vi "testing_cw_sweep.vi"() -> ()   [LabVIEW 2015, in "Tausand AB1000.lvlib"]
uses:
  <instrlib>/Tausand AB1000/Tausand AB1000.lvlib
  <instrlib>/Tausand AB1000/Public/Controls/deviceTypeRing.ctl
  <instrlib>/Tausand AB1000/Public/Controls/counters4ch.ctl
  <instrlib>/Tausand AB1000/Public/Controls/channelRing.ctl
panel:
  in  "device type (any)":T1 items=["any"=0, "AB1002"=1002, "AB1004"=1004, "AB1502"=1502, "AB1504"=1504, "AB1902"=1902, "AB1904"=1904, "AB2002"=2002, "AB2004"=2004, "AB2502"=2502, "AB2504"=2504, "AB2902"=2902, "AB2904"=2904]
  out "tausand values":u32[][](array[numeric])
  in  "delay D (ns)":u32
  in  "delay C (ns)":u32
  in  "delay B (ns)":u32
  in  "delay A (ns)":u32
  out "i case":i32
  out "total cases":i32
  in  "Stop Button":bool
  out "coinc Chart":T2(graph)
  out "current values":T3
  in  "sampling (ms)":u32=1000
  out "i cw":i32
  out "device type":T1 items=["any"=0, "AB1002"=1002, "AB1004"=1004, "AB1502"=1502, "AB1504"=1504, "AB1902"=1902, "AB1904"=1904]
  out "cw array":u32[](array[numeric])
  in  "step cw":u32=1
  in  "max cw":u32=10
  in  "min cw":u32=1
  out "current cw (ns)":u32
  in  "VISA resource name":refnum<visa-resource-name>
  # "case"
  # "out of"
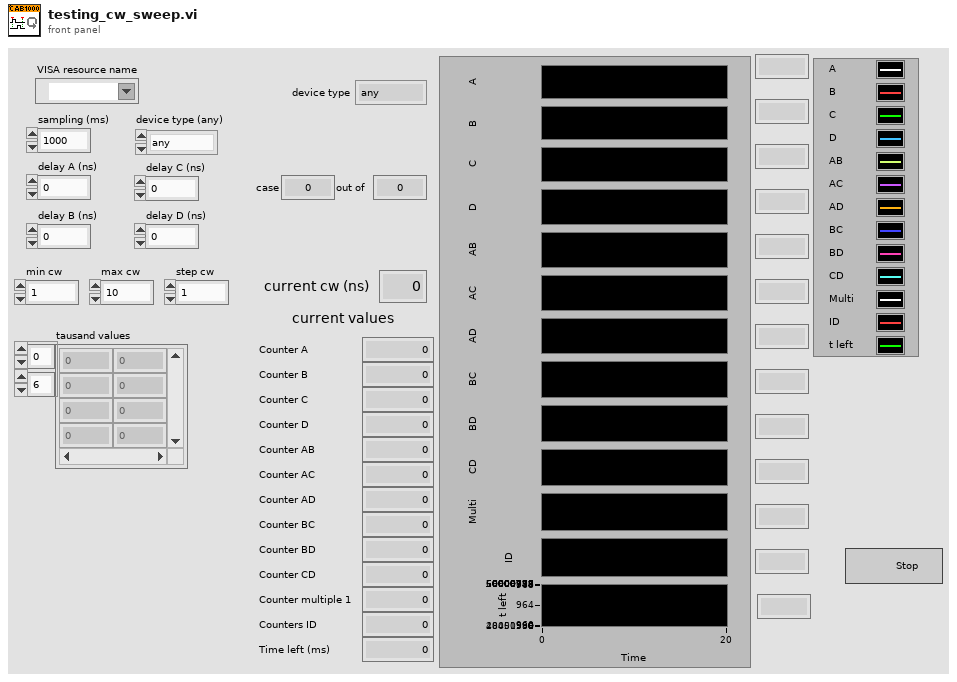
[diagram p1: front panel]
types:
  T1 = typedef "Tausand AB1000.lvlib/deviceTypeRing.ctl" = u16
  T2 = cluster{"counter_A":u32, "counter_B":u32, "counter_C":u32, "counter_D":u32, "counter_AB":u32, "counter_AC":u32, "counter_AD":u32, "counter_BC":u32, "counter_BD":u32, "counter_CD":u32, "counter_multiple_1":u32, "counters_ID":u32, "time_left":u32}
  T3 = typedef "Tausand AB1000.lvlib/counters4ch.ctl" = cluster{"counter_A":u32, "counter_B":u32, "counter_C":u32, "counter_D":u32, "counter_AB":u32, "counter_AC":u32, "counter_AD":u32, "counter_BC":u32, "counter_BD":u32, "counter_CD":u32, "counter_multiple_1":u32, "counters_ID":u32, "time_left":u32}
  T4 = typedef "Tausand AB1000.lvlib/channelRing.ctl" = u8
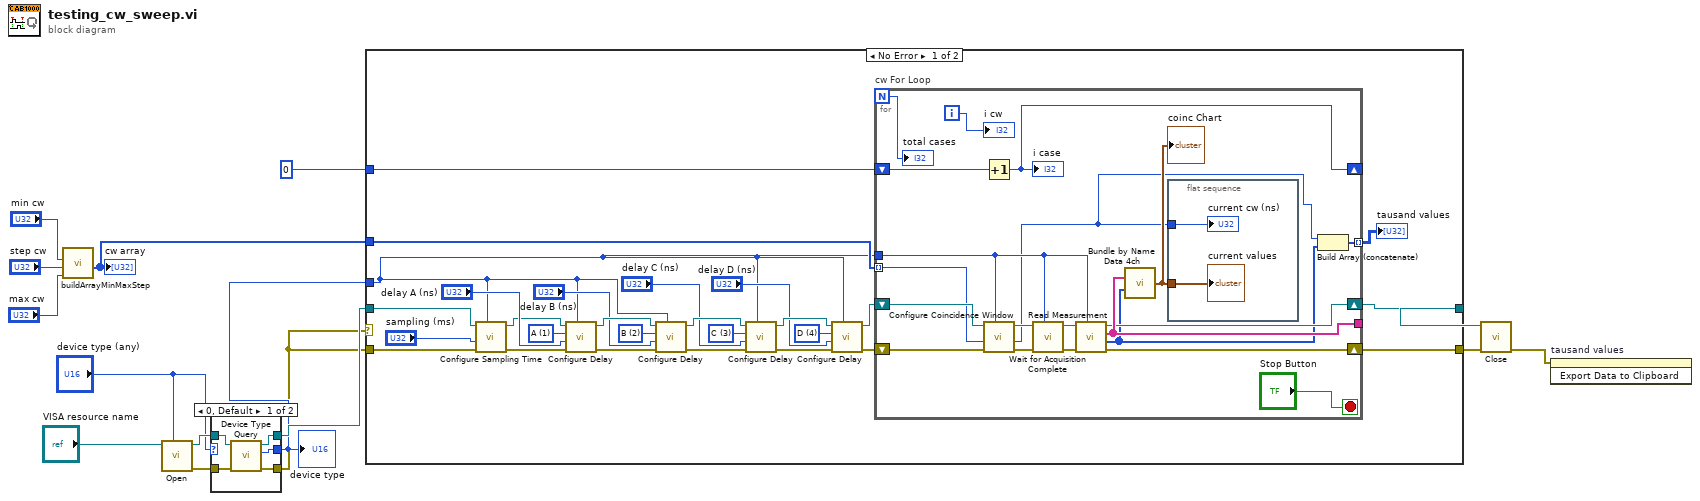
[diagram p0: block diagram]
diagram:
  n1 = call <instrlib>:"buildArrayMinMaxStep.vi"("max (10)"="max cw", "step (1)"="step cw", "min (0)"="min cw") -> ("array"=w11:i32[])  [unwired: 8 in]
  "cw array" <- w11
  n2 = call <instrlib>:"Open.vi"("device type (any)"="device type (any)", "VISA resource name"="VISA resource name") -> ("error out"=w10:errorcluster, "VISA resource name out"=w9:refnum<visa-resource-name>)  [unwired: 8 in]
  n3 = case shown="0, Default" "device type (any)" {
    selector: "device type (any)" -> [_ w22]
    tunnel: w10 -> [w20 w21]
    tunnel: w9 -> [w19 w23]
    tunnel: [w18 w23] -> w8
    tunnel: [w17 w22] -> w7
    tunnel: [w16 w21] -> w4
    frame 0, Default {
      n4 = call <instrlib>:"Device Type Query.vi"("error in (no error)"=w20, "VISA Refnum in"=w19) -> ("error out"=w16:errorcluster, "device type"=w17:T1, "VISA Refnum out"=w18:refnum<visa-resource-name>)  [unwired: 7 in]
    }
    frame 1.. {
    }
  }
  "device type" <- w7
  n5 = case shown="No Error" w4 {
    tunnel: w11 -> [w50 _]
    tunnel: w4 -> [w46 w74]
    tunnel: w8 -> [w47 w73]
    tunnel: w7 -> [w25 _]
    tunnel: [w49 w73] -> w6
    tunnel: [w48 w74] -> w5
    tunnel: 0 ("i delay") -> [w44 _]
    frame No Error {
      w30 = T4 1 items=["none", "A", "B", "C", "D", "E", "F", "G", "H"] ("channel")
      w31 = T4 2 items=["none", "A", "B", "C", "D", "E", "F", "G", "H"] ("channel")
      w32 = T4 3 items=["none", "A", "B", "C", "D", "E", "F", "G", "H"] ("channel")
      w33 = T4 4 items=["none", "A", "B", "C", "D", "E", "F", "G", "H"] ("channel")
      n6 = call <instrlib>:"Configure Sampling Time.vi"("device type"=w25, "error in (no error)"=w46, "value (1000 ms)"="sampling (ms)", "VISA Refnum in"=w47) -> ("error out"=w29:errorcluster, "VISA Refnum out"=w28:refnum<visa-resource-name>)  [unwired: 5 in, 1 out]
      n7 = call <instrlib>:"Configure Delay.vi"("device type"=w25, "error in (no error)"=w29, "value (0 ns)"="delay A (ns)", "channel"=w30, "VISA Refnum in"=w28) -> ("error out"=w39:errorcluster, "VISA Refnum out"=w38:refnum<visa-resource-name>)  [unwired: 4 in, 1 out]
      n8 = call <instrlib>:"Configure Delay.vi"("device type"=w25, "error in (no error)"=w39, "value (0 ns)"="delay B (ns)", "channel"=w31, "VISA Refnum in"=w38) -> ("error out"=w43:errorcluster, "VISA Refnum out"=w42:refnum<visa-resource-name>)  [unwired: 4 in, 1 out]
      n9 = call <instrlib>:"Configure Delay.vi"("device type"=w25, "error in (no error)"=w43, "value (0 ns)"="delay C (ns)", "channel"=w32, "VISA Refnum in"=w42) -> ("error out"=w41:errorcluster, "VISA Refnum out"=w40:refnum<visa-resource-name>)  [unwired: 4 in, 1 out]
      n10 = call <instrlib>:"Configure Delay.vi"("device type"=w25, "error in (no error)"=w41, "value (0 ns)"="delay D (ns)", "channel"=w33, "VISA Refnum in"=w40) -> ("error out"=w26:errorcluster, "VISA Refnum out"=w27:refnum<visa-resource-name>)  [unwired: 4 in, 1 out]
      n11 = for "cw For Loop" {
        N -> [w55]
        tunnel: w50 -> [w54] mode=indexing
        tunnel: w25 -> [w68]
        tunnel: [w67] -> _
        shift-right: [w66] -> w48
        shift-left: w26 -> [w69]
        shift-right: [w65] -> w49
        shift-left: w27 -> [w70]
        shift-right: [w61] -> _
        shift-left: w44 -> [w62]
        tunnel: [w51] -> w24 mode=indexing
        i -> [w63]
        stop <- "Stop Button" stop-if-true
        n12 = Increment(x=w62) -> (x+1=w61:i32)
        "i case" <- w61
        n13 = call <instrlib>:"Configure Coincidence Window.vi"("device type"=w68, "error in (no error)"=w69, "value ns (10ns)"=w54, "VISA Refnum in"=w70) -> ("error out"=w56:errorcluster, "value ns out"=w52:u32, "VISA Refnum out"=w57:refnum<visa-resource-name>)  [unwired: 5 in]
        n14 = call <instrlib>:"Wait for Acquisition Complete.vi"("device type"=w68, "error in (no error)"=w56, "VISA resource name"=w57) -> ("error out"=w60:errorcluster, "VISA resource name out"=w59:refnum<visa-resource-name>)  [unwired: 7 in]
        n15 = call <instrlib>:"Read Measurement.vi"("device type"=w68, "error in (no error)"=w60, "VISA Refnum in"=w59) -> ("error out"=w66:errorcluster, "values"=w53:u32[], "labels"=w67:string[], "VISA Refnum out"=w65:refnum<visa-resource-name>)  [unwired: 3 in, 2 out]
        n16 = call <instrlib>:"Bundle by Name Data 4ch.vi"("names"=w67, "values"=w53) -> ("output cluster 4ch"=w58:T3)  [unwired: 13 in]
        "coinc Chart" <- w58
        n17 = flat-sequence {
          tunnel: w58 -> [w72]
          tunnel: w52 -> [w71]
          frame #0 {
            "current values" <- w72
            "current cw (ns)" <- w71
          }
        }
        n18 = Build Array (concatenate)(w52, w53) -> (w51:u32[])
        "i cw" <- w63
        "total cases" <- w55
      }
      "tausand values" <- w24
    }
    frame Error {
    }
  }
  n19 = call <instrlib>:"Close.vi"("error in (no error)"=w5, "VISA resource name"=w6) -> ("error out"=w2:errorcluster)  [unwired: 9 in]
  n20 = invoke on="tausand values" class="Arr (strict)" method="Export Data to Clipboard"(error in=w2) -> ()  [unwired: 2 in, 3 out]
